vi "endCanon.vi"(8 "error in":errorcluster, 11 "reason":i32) -> (0 "error out":errorcluster)   [LabVIEW 2013]
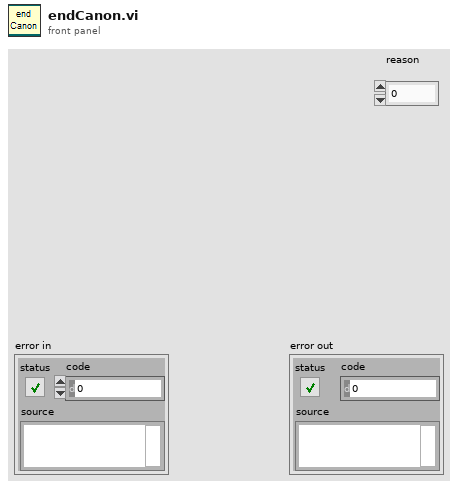
[diagram p1: front panel]
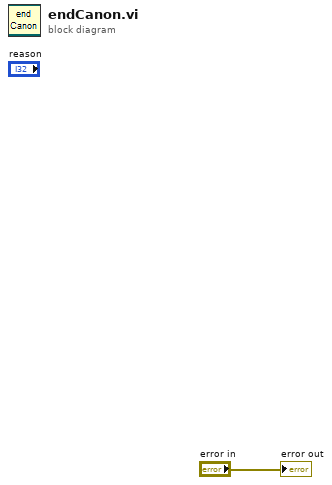
[diagram p0: block diagram]
diagram:
  "error out" <- "error in"
